vi "test.vi"() -> ()   [LabVIEW 2012]
uses:
  Autofocus/Autofocus.lvclass
  Autofocus/Sharpness Measure.ctl
panel:
  in  "Sharpness measure":T1
  in  "File Path":path
  out "sharpness out":dbl
  out "Autofocus out":refnum<class "Autofocus.lvclass">
  in  "Autofocus in":refnum<class "Autofocus.lvclass">
  out "double precision float":dbl[][](array[numeric])
  in  "error in (no error)":errorcluster
  out "error out":errorcluster
  out "Image Source":T2(plugin-control)
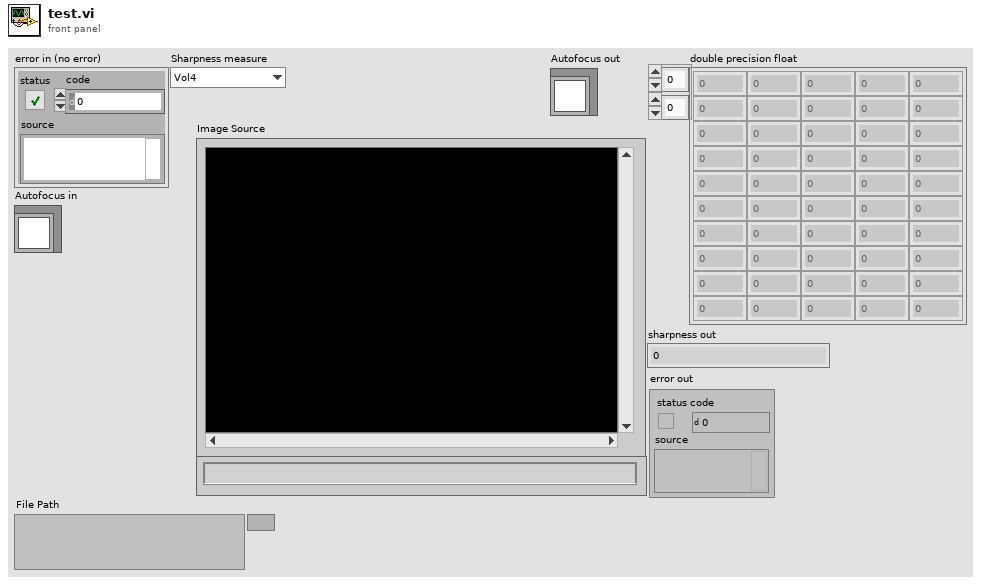
[diagram p1: front panel]
types:
  T1 = typedef "Autofocus.lvclass/Sharpness Measure.ctl" = enum16{"Vol4", "Gradient Square"}
  T2 = typedef "IMAQ Image.ctl" = refnum<image>
  T3 = typedef "Image Type" = u32
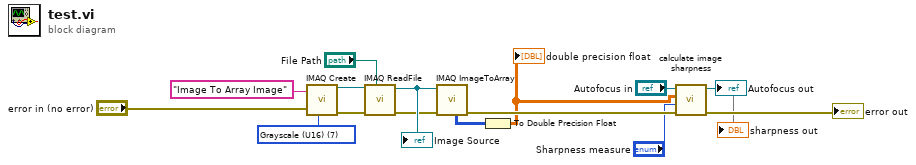
[diagram p0: block diagram]
diagram:
  w14 = T3 7 items=["Grayscale (U8)", "Grayscale (I16)", "Grayscale (SGL)", "Complex (CSG)", "RGB (U32)", "HSL (U32)", "RGB (U64)", "Grayscale (U16)"] ("Image Type")
  n1 = call "IMAQ Create"("Image Name"="Image To Array Image", "Image Type"=w14, "error in (no error)"="error in (no error)") -> ("New Image"=w13:T2, "error out"=w12:errorcluster)  [unwired: 2 in]
  n2 = call "IMAQ ReadFile"("File Path"="File Path", "error in (no error)"=w12, "Image"=w13) -> ("error out"=w15:errorcluster, "Image Out"=w16:T2)  [unwired: 4 in, 3 out]
  "Image Source" <- w16
  n3 = call "IMAQ ImageToArray"("error in (no error)"=w15, "Image"=w16) -> ("Image Pixels (U16)"=w9:u16[][], "error out"=w6:errorcluster)  [unwired: 2 in, 3 out]
  n4 = To Double Precision Float(number=w9) -> (double precision float=w4:dbl[][])
  "double precision float" <- w4
  n5 = call-dynamic "calculate image sharpness.vi"("error in (no error)"=w6, "Sharpness measure"="Sharpness measure", 10:w4, "Autofocus in"="Autofocus in") -> ("error out"=→"error out":errorcluster, 2:→"sharpness out", "Autofocus out"=→"Autofocus out":refnum<class "Autofocus.lvclass">)  [unwired: 5 in]
